vi "Retrieve Data From FPGA.vi"(8 "error in (no error)":errorcluster, 11 "FPGA VI Reference In":refnum<k20>) -> (0 "error out":errorcluster)   [LabVIEW 2016]
uses:
  Typedefs/Monitor Data Operation.ctl
  Typedefs/LV2G Operation.ctl
  Typedefs/IO Buffer Operation.ctl
  <vilib>/Utility/error.llb/Error Cluster From Error Code.vi
  <vilib>/rvi/errors/niLvFpgaAdjustHostInterfaceError.vi
  <vilib>/rvi/interface/nirviMethod/nirviMethod.xnode
  <vilib>/FPGAPlugInAG/Dynamic/niLvFpga_ReadFifo_Dynamic.vi
  <vilib>/rvi/errors/niLvFpgaMergeErrorWithErrorCode.vi
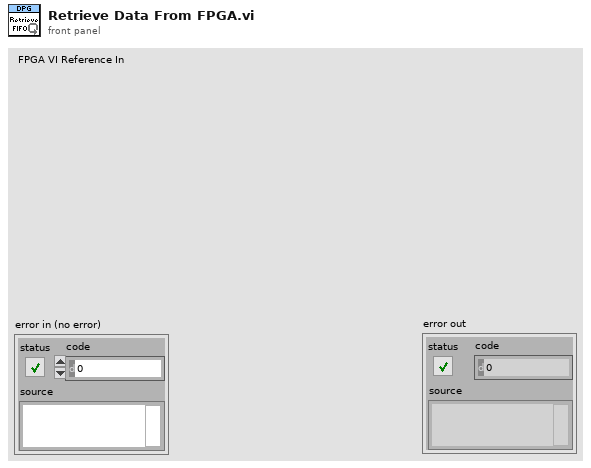
[diagram p1: front panel]
types:
  T1 = typedef "Monitor Data Operation.ctl" = enum16{"Obtain", "Enqueue", "Read Elements", "Flush", "Release", "Read Last Element"}
  T2 = typedef "LV2G Operation.ctl" = enum16{"Initialize", "Set", "Get", "Close"}
  T3 = typedef "IO Buffer Operation.ctl" = enum16{"Initialize", "Write IO Data_Rd", "Read IO Data_Rd", "Write IO Data_Wr", "Read IO Data_Wr", "Write  IO Data_Dir", "Read  IO Data_Dir", "Write Host to Target FIFO", "Read Host to Target FIFO", "Write Target to Host FIFO", "Read Target to Host FIFO", "Write Monitor Enable?", "Read Monitor Enable?", "Close"}
  T4 = typedef "Monitor Data Element.ctl" = cluster{"Pin Data":u32, "Transition ":u32}
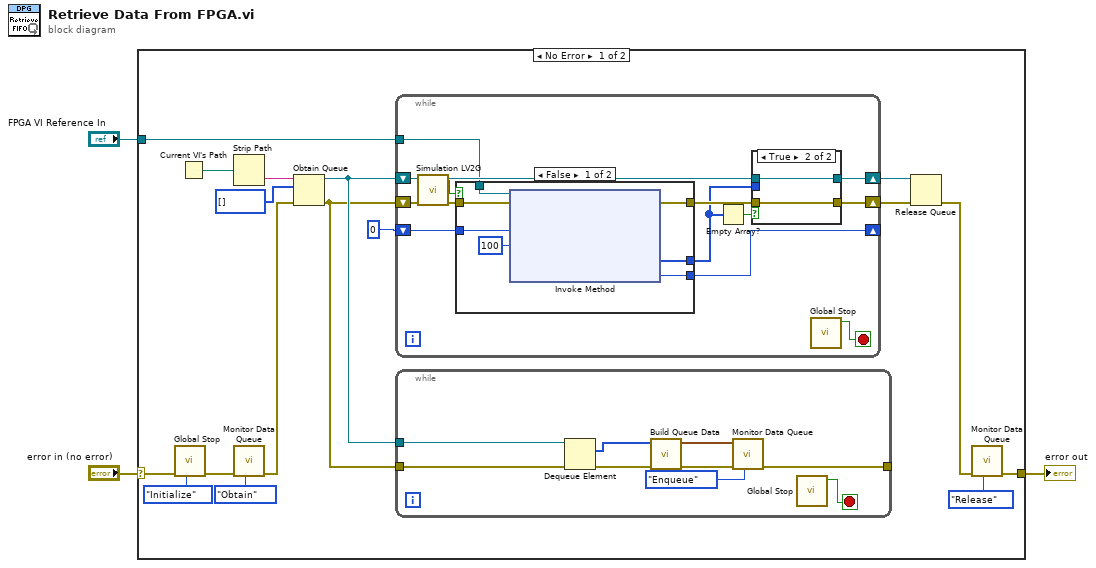
[diagram p0: block diagram]
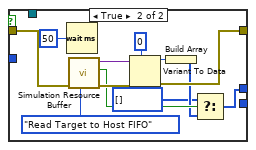
[diagram p2: hidden frame]
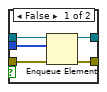
[diagram p3: hidden frame]
diagram:
  n1 = case shown="No Error" "error in (no error)" {
    selector: "error in (no error)" -> [w8 w69]
    tunnel: "FPGA VI Reference In" -> [w16 _]
    tunnel: [w5 w69] -> w1
    frame No Error {
      n2 = call "Global Stop.vi"("Stop Operation (Get)"=LV2G_Operation."Initialize", "error in (no error)"=w8) -> ("error out"=w9:errorcluster)  [unwired: 8 in, 1 out]
      n3 = Current VI's Path() -> (path=w14:path)
      n4 = Strip Path(path=w14) -> (name=w15:string)  [unwired: 1 out]
      n5 = call "Monitor Data Queue.vi"("Queue Function"=Monitor_Data_Operation."Obtain", "error in (no error)"=w9) -> ("error out"=w11:errorcluster)  [unwired: 6 in, 3 out]
      n6 = Obtain Queue(name (unnamed)=w15, element data type=u64[] [], error in (no error)=w11) -> (queue out=w18:refnum<queue>, error out=w17:errorcluster)  [unwired: 2 in, 1 out]
      n7 = while {
        shift-right: [w41] -> _
        shift-left: u32 0 ("Number of Elements") -> [w42]
        shift-right: [w38] -> w13
        shift-left: w17 -> [w32]
        tunnel: w16 -> [w35]
        shift-right: [w34] -> w12
        shift-left: w18 -> [w40]
        stop <- w33 stop-if-true
        n8 = call "Simulation LV2G.vi"("error in (no error)"=w32) -> ("error out"=w31:errorcluster, "Simulation? out"=w30:bool)  [unwired: 9 in]
        n9 = case shown="False" w30 {
          tunnel: w31 -> [w49 w61]
          tunnel: w42 -> [w48 _]
          tunnel: [w47 _] -> w41
          tunnel: [w45 w57] -> w39
          tunnel: [w44 w51] -> w37
          tunnel: w35 -> [w43 _]
          frame False {
            n10 = xnode "Invoke Method"("FPGA VI Reference In"=w43, "error in"=w49, "Number of Elements"=w48, "Timeout (ms)"=100) -> ("error out"=w45:errorcluster, "Data"=w44:u64[], "Elements Remaining"=w47:u32)  [unwired: 1 out]
          }
          frame True {
            n11 = Wait (ms)(milliseconds to wait=u32 50) -> ()  [unwired: 1 out]
            n12 = call "Simulation Resource Buffer.vi"("IO Buffer Operation"=IO_Buffer_Operation."Read Target to Host FIFO", "error in (no error)"=w61) -> ("error out"=w59:errorcluster, "Timed Out?"=w54:bool, "Data out"=w58:variant)  [unwired: 7 in]
            n13 = Variant To Data(error in=w59, type=u64 0 ("Elements Remaining"), Variant=w58) -> (data=w55:u64, error out=w57:errorcluster)
            n14 = Build Array(w55) -> (w53:u64[])
            n15 = Select(t=u64[] [], s=w54, f=w53) -> (s? t:f=w51:u64[])
          }
        }
        n16 = Empty Array?(array=w37) -> (empty?=w36:bool)
        n17 = case shown="True" w36 {
          tunnel: w40 -> [w66 w67]
          tunnel: w37 -> [w65 _]
          tunnel: w39 -> [w64 w68]
          tunnel: [w63 w68] -> w38
          tunnel: [w62 w67] -> w34
          frame False {
            n18 = Enqueue Element(queue=w66, element=w65, error in (no error)=w64) -> (queue out=w62:refnum<queue>, error out=w63:errorcluster)  [unwired: 1 in, 1 out]
          }
          frame True {
          }
        }
        n19 = call "Global Stop.vi"() -> ("Stop? out"=w33:bool)  [unwired: 10 in, 1 out]
      }
      n20 = while {
        tunnel: w18 -> [w29]
        tunnel: w17 -> [w28]
        tunnel: [w22] -> _
        stop <- w21 stop-if-true
        n21 = Dequeue Element(queue=w29, error in (no error)=w28) -> (element=w26:u64[], error out=w27:errorcluster)  [unwired: 1 in, 2 out]
        n22 = call "Build Queue Data.vi"("error in (no error)"=w27, "Data from FIFO"=w26) -> ("error out"=w25:errorcluster, "Data to Queue"=w24:T4[])  [unwired: 8 in]
        n23 = call "Monitor Data Queue.vi"("Queue Function"=Monitor_Data_Operation."Enqueue", "error in (no error)"=w25, "Data From FIFO"=w24) -> ("error out"=w22:errorcluster)  [unwired: 5 in, 3 out]
        n24 = call "Global Stop.vi"() -> ("Stop? out"=w21:bool)  [unwired: 10 in, 1 out]
      }
      n25 = Release Queue(queue=w12, error in (no error)=w13) -> (error out=w6:errorcluster)  [unwired: 1 in, 2 out]
      n26 = call "Monitor Data Queue.vi"("Queue Function"=Monitor_Data_Operation."Release", "error in (no error)"=w6) -> ("error out"=w5:errorcluster)  [unwired: 6 in, 3 out]
    }
    frame Error {
    }
  }
  "error out" <- w1
